vi "Freeze Value Boolean.vi"(1 "input":bool, 4 "Freeze Value":bool=TRUE) -> (21 "output":bool)   [LabVIEW 2019, in "Untitled Library 1.lvlib"]
uses:
  Untitled Library 1.lvlib
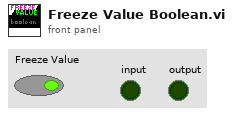
[diagram p1: front panel]
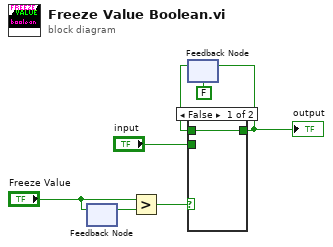
[diagram p0: block diagram]
diagram:
  n1 = feedback #1() -> (w7:bool)  [unwired: 1 in]
  n2 = feedback-in #1("Freeze Value") -> ()
  n3 = Greater?(x="Freeze Value", y=w7) -> (0:w5:bool)
  n4 = feedback #2(FALSE ("input")) -> (w4:bool)
  n5 = case shown="False" w5 {
    tunnel: [w8 w9] -> w2
    tunnel: w4 -> [w8 _]
    tunnel: "input" -> [_ w9]
    frame False {
    }
    frame True {
    }
  }
  "output" <- w2
  n6 = feedback-in #2(w2) -> ()
